vi "constrain derivative.vi"(0 "Accel":dbl, 1 "dt":dbl, 5 "Velo":dbl, 7 "velo unit":dbl, 9 "Accel max constant":dbl, 11 "Velo max constant":dbl, 12 "Jerk max constant":dbl) -> (4 "Velo Out":dbl)   [LabVIEW 2014]
panel:
  out "velo min":dbl
  out "velo max":dbl
  out "max accel":dbl
  out "min accel":dbl
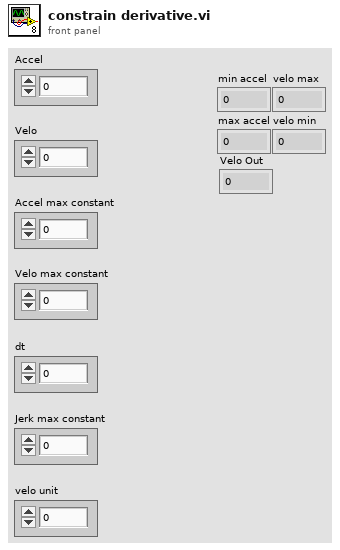
[diagram p1: front panel]
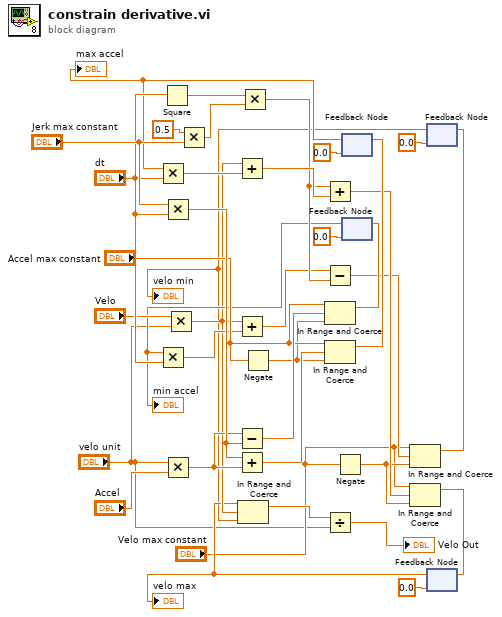
[diagram p0: block diagram]
diagram:
  n1 = Square(x="dt") -> (x^2=w24:dbl)
  n2 = Multiply(x="Jerk max constant", y="dt") -> (x*y=w34:dbl)
  n3 = Multiply(x="velo unit", y="Accel") -> (x*y=w12:dbl)
  n4 = Multiply(x="Velo", y="velo unit") -> (x*y=w5:dbl)
  n5 = Multiply(x=0.5, y="Jerk max constant") -> (x*y=w25:dbl)
  n6 = Subtract(x=w12, y=w34) -> (x-y=w33:dbl)
  n7 = Add(x=w34, y=w12) -> (x+y=w37:dbl)
  n8 = Multiply(x=w24, y=w25) -> (x*y=w19:dbl)
  n9 = Negate(x="Accel max constant") -> (-x=w31:dbl)
  n10 = In Range and Coerce(upper limit="Accel max constant", x=w33, lower limit=w31) -> (coerced(x)=w29:dbl)  [unwired: 1 out]
  n11 = In Range and Coerce(upper limit="Accel max constant", x=w37, lower limit=w31) -> (coerced(x)=w36:dbl)  [unwired: 1 out]
  n12 = Negate(x="Velo max constant") -> (-x=w17:dbl)
  n13 = feedback-in #1(w36) -> ()
  n14 = feedback #1(0.0 ("Accel")) -> (w6:dbl)
  "max accel" <- w6
  n15 = Multiply(x=w6, y="dt") -> (x*y=w28:dbl)
  n16 = Add(x=w5, y=w28) -> (x+y=w20:dbl)
  n17 = Add(x=w19, y=w20) -> (x+y=w22:dbl)
  n18 = feedback #2(0.0 ("Accel")) -> (w7:dbl)
  "min accel" <- w7
  n19 = Multiply(x=w7, y="dt") -> (x*y=w10:dbl)
  n20 = Add(x=w5, y=w10) -> (x+y=w8:dbl)
  n21 = Subtract(x=w8, y=w19) -> (x-y=w18:dbl)
  n22 = feedback-in #2(w29) -> ()
  n23 = In Range and Coerce(upper limit="Velo max constant", x=w18, lower limit=w17) -> (coerced(x)=w15:dbl)  [unwired: 1 out]
  n24 = In Range and Coerce(upper limit="Velo max constant", x=w22, lower limit=w17) -> (coerced(x)=w21:dbl)  [unwired: 1 out]
  n25 = feedback #3(0.0) -> (w3:dbl)
  "velo min" <- w3
  n26 = feedback-in #3(w15) -> ()
  n27 = feedback-in #4(w21) -> ()
  n28 = feedback #4(0.0) -> (w4:dbl)
  "velo max" <- w4
  n29 = In Range and Coerce(upper limit=w4, x=w5, lower limit=w3) -> (coerced(x)=w14:dbl)  [unwired: 1 out]
  n30 = Divide(x=w14, y="velo unit") -> (x/y=→"Velo Out":dbl)
